vi "Grapher_Create.vi"(0 "reference in":refnum<class "Grapher.lvclass">, 1 "Indicator Refs":T1, 2 "Update Rate (ms)":i32=50, 4 "Power Module":refnum<class "PowerModuleInterface.lvclass">, 5 "Error In":errorcluster) -> (14 "reference out":refnum<class "Grapher.lvclass">, 19 "Error Out":errorcluster)   [LabVIEW 2023, in "Grapher.lvclass"]
uses:
  Grapher.lvclass
  Types/Indicators.ctl
  builds/PowerModuleInterface/PowerModuleInterface.lvlibp/Classes/PowerModule_interface/PowerModuleInterface.lvclass
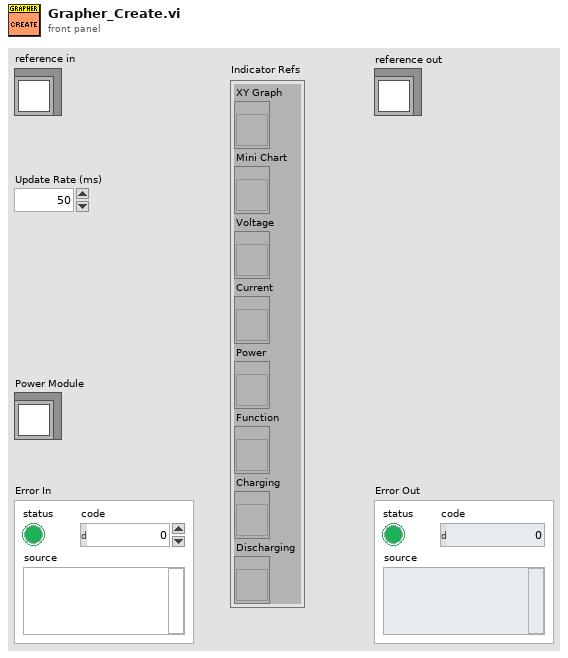
[diagram p1: front panel]
types:
  T1 = typedef "Indicators.ctl" = cluster{"XY Graph":refnum<vi>, "Mini Chart":refnum<vi>, "Voltage":refnum<vi>, "Current":refnum<vi>, "Power":refnum<vi>, "Function":refnum<vi>, "Charging":refnum<vi>, "Discharging":refnum<vi>}
  T2 = typedef "Grapher.lvclass/ObjectAttributes.ctl" = cluster{"Indicator Refs":T1, "Update Rate (ms)":i32, "Power Module":refnum<class "PowerModuleInterface.lvclass">}
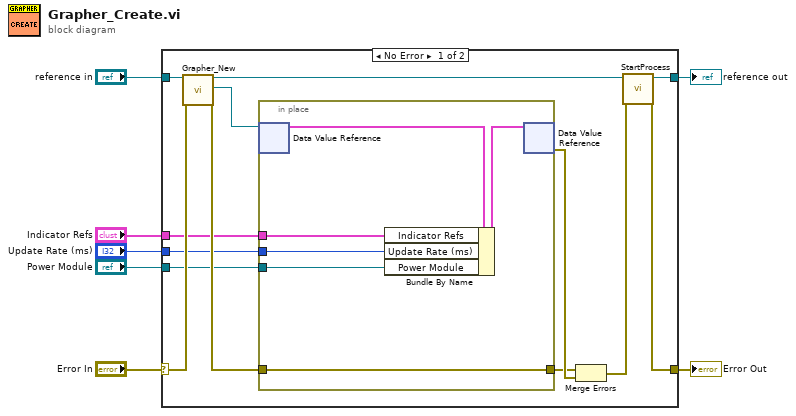
[diagram p0: block diagram]
diagram:
  n1 = case shown="No Error" "Error In" {
    selector: "Error In" -> [w19 w28]
    tunnel: [w11 w28] -> w6
    tunnel: "reference in" -> [w20 w27]
    tunnel: [w13 w27] -> w4
    tunnel: "Indicator Refs" -> [w10 _]
    tunnel: "Update Rate (ms)" -> [w9 _]
    tunnel: "Power Module" -> [w8 _]
    frame No Error {
      n2 = call "Grapher_New.vi"("reference in"=w20, "Error In"=w19) -> ("reference out"=w14:refnum<class "Grapher.lvclass">, "DVRRefOut"=w17:refnum<data-value>, "Error Out"=w16:errorcluster)  [unwired: 14 in, 1 out]
      n3 = in-place {
        in-place-border: w16 -> [w24]
        in-place-border: [w24] -> w15
        in-place-border: w10 -> [w23]
        in-place-border: w9 -> [w22]
        in-place-border: w8 -> [w21]
        n4 = in-place-dvr #1(w17) -> (w25:T2)  [unwired: 1 out]
        n5 = Bundle By Name(cluster=w25, "Indicator Refs"=w23, "Update Rate (ms)"=w22, "Power Module"=w21) -> (w26:T2)
        n6 = in-place-dvr #1(w26) -> (w18:errorcluster)  [unwired: 1 out]
      }
      n7 = Merge Errors(w15, w18) -> (w12:errorcluster)
      n8 = call "StartProcess.vi"("reference in"=w14, "Error In"=w12) -> ("reference out"=w13:refnum<class "Grapher.lvclass">, "Error Out"=w11:errorcluster)  [unwired: 14 in, 2 out]
    }
    frame Error {
      # "VI-TechBaseTemplate_Simple_6x8x6"
    }
  }
  "Error Out" <- w6
  "reference out" <- w4
